vi "meth.SetDebug.vi"(0 "class.GLue in":refnum<class "class.GLue.lvclass">, 7 "Enable":i32, 11 "error in":errorcluster, 13 "ms timeout (-1)":i32=-1) -> (4 "class.GLue out":refnum<class "class.GLue.lvclass">, 15 "error out":errorcluster)   [LabVIEW 2014, in "GLue.lvlib" / "class.GLue.lvclass"]
uses:
  class.GLue.lvclass
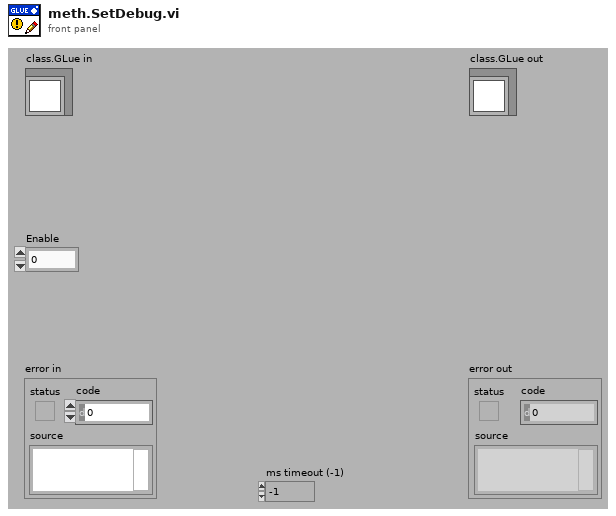
[diagram p1: front panel]
types:
  T1 = typedef "Semaphore RefNum" = refnum<k1>
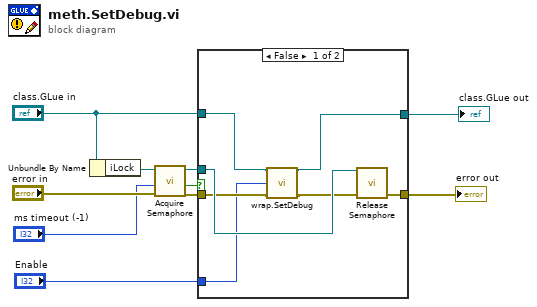
[diagram p0: block diagram]
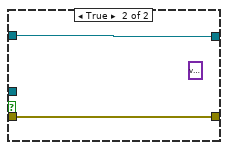
[diagram p2: hidden frame]
diagram:
  n1 = Unbundle By Name("class.GLue in") -> ("iLock"=w10:T1)
  n2 = call <vilib>:"Acquire Semaphore.vi"("error in (no error)"="error in", "ms timeout (-1)"="ms timeout (-1)", "semaphore"=w10) -> ("error out"=w9:errorcluster, "timed out"=w8:bool, "semaphore out"=w7:T1)  [unwired: 2 in]
  n3 = case shown="False" w8 {
    tunnel: [w17 w18] -> w2
    tunnel: [w14 w19] -> w3
    tunnel: "class.GLue in" -> [w15 w19]
    tunnel: w9 -> [w13 w18]
    tunnel: w7 -> [w16 _]
    tunnel: "Enable" -> [w11 _]
    frame False {
      n4 = call "wrap.SetDebug.vi"("class.GLue in"=w15, "Enable"=w11, "error in (no error)"=w13) -> ("class.GLue out"=w14:refnum<class "class.GLue.lvclass">, "error out"=w12:errorcluster)  [unwired: 11 in]
      n5 = call <vilib>:"Release Semaphore.vi"("error in (no error)"=w12, "semaphore"=w16) -> ("error out"=w17:errorcluster)  [unwired: 4 in, 1 out]
    }
    frame True {
      (unwired) variant ("Data out")
    }
  }
  "error out" <- w2
  "class.GLue out" <- w3
